vi "Should Stop.vi"(11 "Exit App.lvclass":refnum<class "Exit App.lvclass">) -> (2 "stop?":bool)   [LabVIEW 2010, in "Exit App.lvclass"]
doc: "Exit App.lvclass is the only child class of Application Command.lvclass that overwrites Should Stop.vi. For this instance, the value of the stop? output is set to TRUE. \n\nThe other classes do not need to overwrite this method since they will always pass a value of FALSE, as defined in Application Command.lvclass."
uses:
  Exit App.lvclass
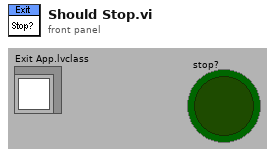
[diagram p1: front panel]
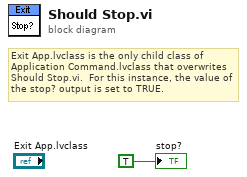
[diagram p0: block diagram]
diagram:
  # "Exit App.lvclass is the only child class of \nApplication Command.lvclass that overwrites \nShould Stop.vi.  For this instance, the value of \nthe stop? output is set to TRUE."
  "stop?" <- TRUE ("stop?")
